vi "Read Data.vi"(8 "error in (no error)":errorcluster, 11 "CS++MCS in":refnum<class "CS++MCS.lvclass">) -> (0 "error out":errorcluster, 2 "Waveform Data":waveform(dbl), 3 "CS++MCS out":refnum<class "CS++MCS.lvclass">)   [LabVIEW 2015, in "CS++MCS.lvlib" / "CS++MCS.lvclass"]
doc: "This VI reads out the MCS device and returns the aqcuired waveform."
uses:
  CS++MCS.lvclass
  CSPP_Core/Classes/CS++ProcessVariables/ProcessVariable/PV.lvclass
  PV-Enum.ctl
  CSPP_Core/Classes/CS++ProcessVariables/ProcessVariable/PV.lvclass/PV.ctl
  CS++MCS.lvclass/CS++MCS.ctl
  CSPP_Core/Classes/CS++ProcessVariables/ProcessVariable/Write Data.vi
  CSPP_Core/Classes/CS++ProcessVariables/ProcessVariable/Write Timestamp.vi
  CSPP_Core/Classes/CS++ProcessVariables/ProcessVariable/Write Quality.vi
  CSPP_Core/Classes/CS++ProcessVariables/ProcessVariable/Write status.vi
  CSPP_Core/Classes/CS++ProcessVariables/PVConnection/PVConnection.lvclass
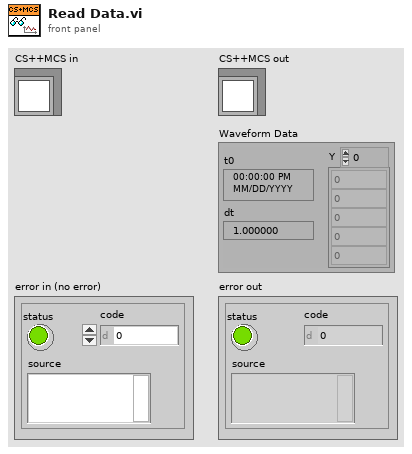
[diagram p1: front panel]
types:
  T1 = typedef "CS++MCS.lvlib/CS++MCS.lvclass/PV-Enum.ctl" = enum16{"Counts/I32", "TotalCounts/I32", "Status/I8", "BinWidth/Dbl", "NofBins/I32", "NofRecords /I32", "DiscLvl/Dbl", "TrigLvl/Dbl", "DiscSlope/U16", "TrigSlope/U16", "ActWaveform/AWfm|0:1"}
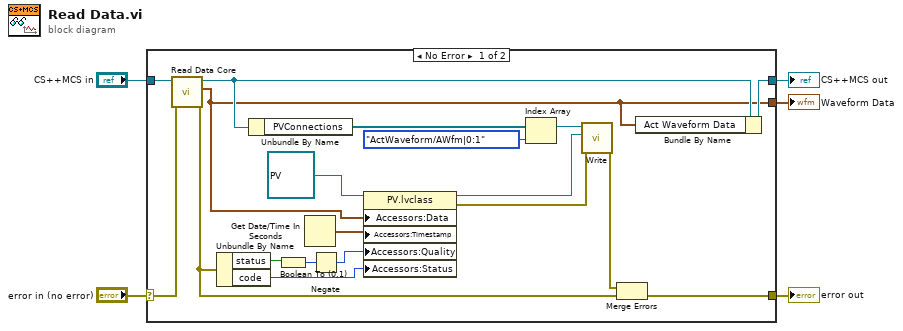
[diagram p0: block diagram]
diagram:
  n1 = case shown="No Error" "error in (no error)" {
    selector: "error in (no error)" -> [w23 w26]
    tunnel: [w7 w26] -> w4
    tunnel: [w10 w25] -> w2
    tunnel: "CS++MCS in" -> [w24 w25]
    tunnel: [w9 _] -> w1
    frame No Error {
      n2 = call-dynamic "Read Data Core.vi"("error in (no error)"=w23, "CS++MCS in"=w24) -> ("error out"=w8:errorcluster, "Waveform Data"=w9:waveform(dbl), "CS++MCS out"=w11:refnum<class "CS++MCS.lvclass">)  [unwired: 7 in]
      n3 = Unbundle By Name(w8) -> ("status"=w20:bool, "code"=w17:i32)
      n4 = Unbundle By Name(w11) -> ("PVConnections"=w22:refnum<class "PVConnection.lvclass">[])
      n5 = Boolean To (0,1)(Boolean=w20) -> (0, 1=w19:i16)
      n6 = Get Date/Time In Seconds() -> (seconds since 1Jan1904=w14:timestamp)
      n7 = Negate(x=w19) -> (-x=w18:i16)
      n8 = property class="PV.lvclass"(reference=refnum<class "PV.lvclass"> refnum ("CS++ProcessVariables.lvlib:PV.lvclass"), "Accessors:Data"=w9, "Accessors:Timestamp"=w14, "Accessors:Quality"=w18, "Accessors:Status"=w17) -> (reference out=w15:refnum<class "PV.lvclass">, error out=w16:errorcluster)  [unwired: 1 in]
      n9 = Index Array(array=w22, index=PV-Enum."ActWaveform/AWfm|0:1" ("PV-Enum")) -> (element=w13:refnum<class "PVConnection.lvclass">)
      n10 = call "Write.vi"("error in (no error)"=w16, "PV"=w15, "PVConnection in"=w13) -> ("error out"=w6:errorcluster)  [unwired: 7 in, 1 out]
      n11 = Merge Errors(w6, w8) -> (w7:errorcluster)
      n12 = Bundle By Name(cluster=w11, "Act Waveform Data"=w9) -> (w10:refnum<class "CS++MCS.lvclass">)
    }
    frame Error {
    }
  }
  "error out" <- w4
  "CS++MCS out" <- w2
  "Waveform Data" <- w1
